vi "Filter Graves.vi"(8 "Error In":errorcluster, 11 "GObjects":refnum<vi>[](array[refnum])) -> (0 "Error Out":errorcluster, 3 "Graves":refnum<vi>[](array[refnum]))   [LabVIEW 2017, in "Toolkit.lvlib"]
doc: "Filters an array of GObject references and keeps only references to graves. Any references that are NOT to a grave are closed."
uses:
  Toolkit.lvlib
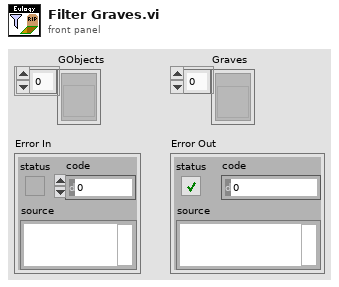
[diagram p1: front panel]
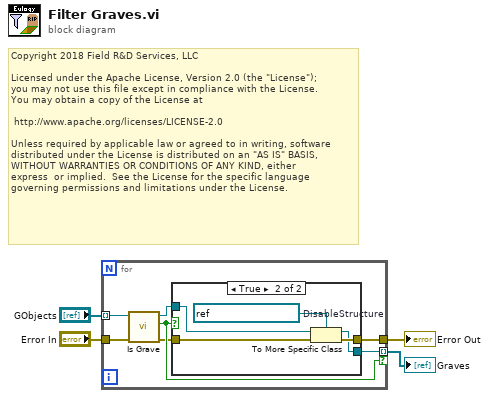
[diagram p0: block diagram]
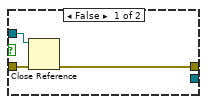
[diagram p2: hidden frame]
diagram:
  # "Copyright 2018 Field R&D Services, LLC\n\nLicensed under the Apache License, Version 2.0 (the \"License\");\nyou may not use this file except in compliance with the License.\nYou may obtain a copy of the License at\n\n\thttp://www.apache.org/licenses/LICENSE-2.0\n\nUnless required by applicable law or agreed to in writing, software\ndistributed under the License is distributed on an \"AS IS\" BASIS,\nWITHOUT WARRANTIES OR CONDITIONS OF ANY KIND, either \nexpress  or implied.  See the License for the specific language \ngoverning permissions and limitations under the License."
  n1 = for {
    tunnel: [w7] -> w3 mode=indexing if=w10
    tunnel: [w8] -> w4
    tunnel: "GObjects" -> [w6] mode=indexing
    tunnel: "Error In" -> [w5]
    n2 = call "Is Grave.vi"("Error In"=w5, "GObject In"=w6) -> ("Error Out"=w9:errorcluster, "Grave?"=w10:bool, "GObject Out"=w11:refnum<vi>)  [unwired: 7 in]
    n3 = case shown="True" w10 {
      tunnel: w11 -> [w14 w19]
      tunnel: w9 -> [w13 w18]
      tunnel: [w12 w16] -> w8
      tunnel: [_ w15] -> w7
      frame False {
        n4 = Close Reference(reference=w14, error in (no error)=w13) -> (error out=w12:errorcluster)
      }
      frame True {
        w17 = refnum<vi> refnum  # DisableStructure
        n5 = To More Specific Class(target class=w17, reference=w19, error in=w18) -> (specific class reference=w15:refnum<vi>, error out=w16:errorcluster)
      }
    }
  }
  "Error Out" <- w4
  "Graves" <- w3
